vi "Fetch Single Record Multiple Channel(DBL).vi"(5 "FIFO Type":enum16{"FPGA to Host FIFO (U64)", "Generic"}(ring), 7 "Timeout (s)":i32=5, 8 "error in":errorcluster, 11 "FPGA VI Reference In":refnum<k20>) -> (0 "error out":errorcluster, 2 "Acquired Data":dbl[][](array[numeric]) format="%.2f", 3 "FPGA VI Reference Out":refnum<k20>)   [LabVIEW 2012]
uses:
  <userlib>/FlexRIO Host Library/FlexRIO Host API/Acquire/Fetch/Fetch Acquired Data (U64).vi
  <vilib>/Utility/error.llb/Error Cluster From Error Code.vi
  <vilib>/rvi/errors/niLvFpgaAdjustHostInterfaceError.vi
  <vilib>/rvi/interface/nirviReadWriteControl/nirviReadWriteControl.xnode
  <userlib>/FlexRIO Host Library/FlexRIO Host Library (User).lvlib
  NiFpgaLv.dll
  <vilib>/rvi/interface/Simulation/niFpgaSimulationCallBeginRW.vi
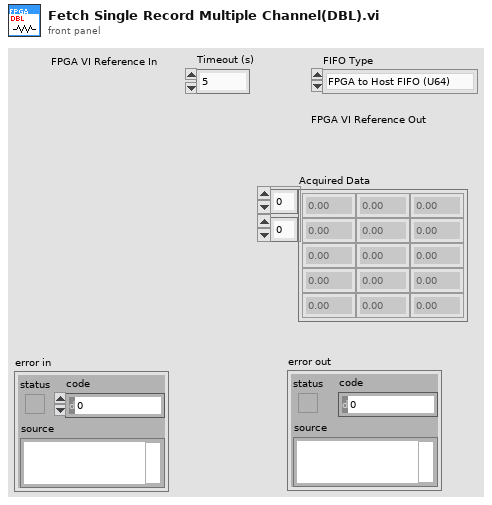
[diagram p1: front panel]
types:
  T1 = cluster{"Load Record Parameters?":bool, "Pre Trigger Samples":u16, "Samples per Record":u16, "Trigger Hold Off":u16, "Record Count":u16}
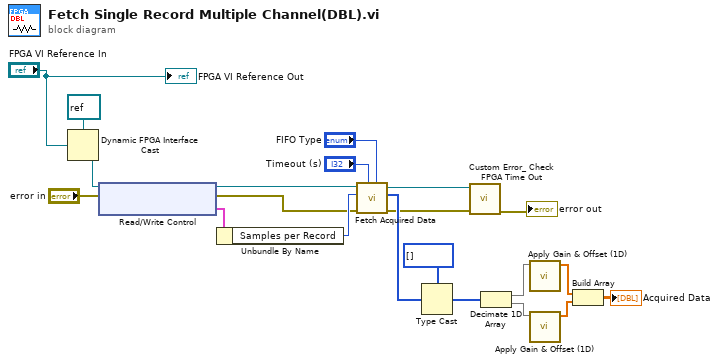
[diagram p0: block diagram]
diagram:
  n1 = Dynamic FPGA Interface Cast(Session In=refnum<k20> refnum ("Type"), Type="FPGA VI Reference In") -> (Session Out=w18:refnum<k20>)
  n2 = xnode "Read/Write Control"("FPGA VI Reference In"=w18, "error in"="error in") -> ("FPGA VI Reference Out"=w15:refnum<k20>, "error out"=w14:errorcluster, "Record Parameters"=w17:T1)
  n3 = Unbundle By Name(w17) -> ("Samples per Record"=w16:u16)
  n4 = call-poly <userlib>:"Fetch Acquired Data.vi"("FIFO Type"="FIFO Type", "Timeout (s)"="Timeout (s)", "error out"=w14, "Samples"=w16, "FPGA Reference In"=w15) -> ("error out"=w6:errorcluster, "Data"=w11:u64[], "FPGA Reference Out"=w7:refnum<k20>)  [unwired: 3 in, 1 out]
  n5 = Type Cast(type=i16[] [], x=w11) -> (*(type *) &x=w12:i16[])
  n6 = call <userlib>:"Custom Error_ Check FPGA Time Out.vi"("error in"=w6, "FPGA VI Reference In"=w7) -> ("error out"=→"error out":errorcluster)  [unwired: 8 in, 1 out]
  n7 = Decimate 1D Array(w12) -> (w4:i16[], w1:i16[])
  n8 = call <userlib>:"Apply Gain & Offset (1D).vi"("Raw Data"=w4) -> ("Scaled Data"=w3:dbl[])  [unwired: 10 in]
  n9 = call <userlib>:"Apply Gain & Offset (1D).vi"("Raw Data"=w1) -> ("Scaled Data"=w2:dbl[])  [unwired: 10 in]
  n10 = Build Array(w3, w2) -> (→"Acquired Data":dbl[][])
  "FPGA VI Reference Out" <- "FPGA VI Reference In"
